vi "getTSRnumber.vi"(8 "error in (no error)":errorcluster, 11 "reference in":refnum<class "File Controller.lvclass">) -> (0 "error out":errorcluster, 3 "reference out":refnum<class "File Controller.lvclass">)   [LabVIEW 2016, in "File Controller.lvclass"]
uses:
  File Controller.lvclass
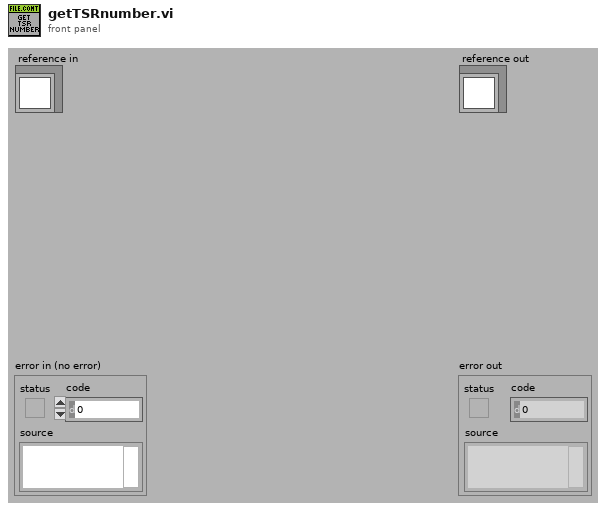
[diagram p1: front panel]
types:
  T1 = typedef "File Controller.lvclass/ObjectAttributesRef.ctl" = refnum<data-value>
  T2 = typedef "File Controller.lvclass/ObjectAttributes.ctl" = cluster{"MyAttribute":dbl, "excelFile_refs":refnum<class "excelFile.lvclass">[], "filePaths":path[], "outlookTemplatePaths":path[], "attachmentTemplatePaths":path[], "configFilePath":path, "not_setting":bool[], "python_ref":refnum<class "python.lvclass">, "TSR":cluster{"number":string, "TSR_path":path, "service_path":path, "email_to":string}}
  T3 = cluster{"number":string, "TSR_path":path, "service_path":path, "email_to":string}
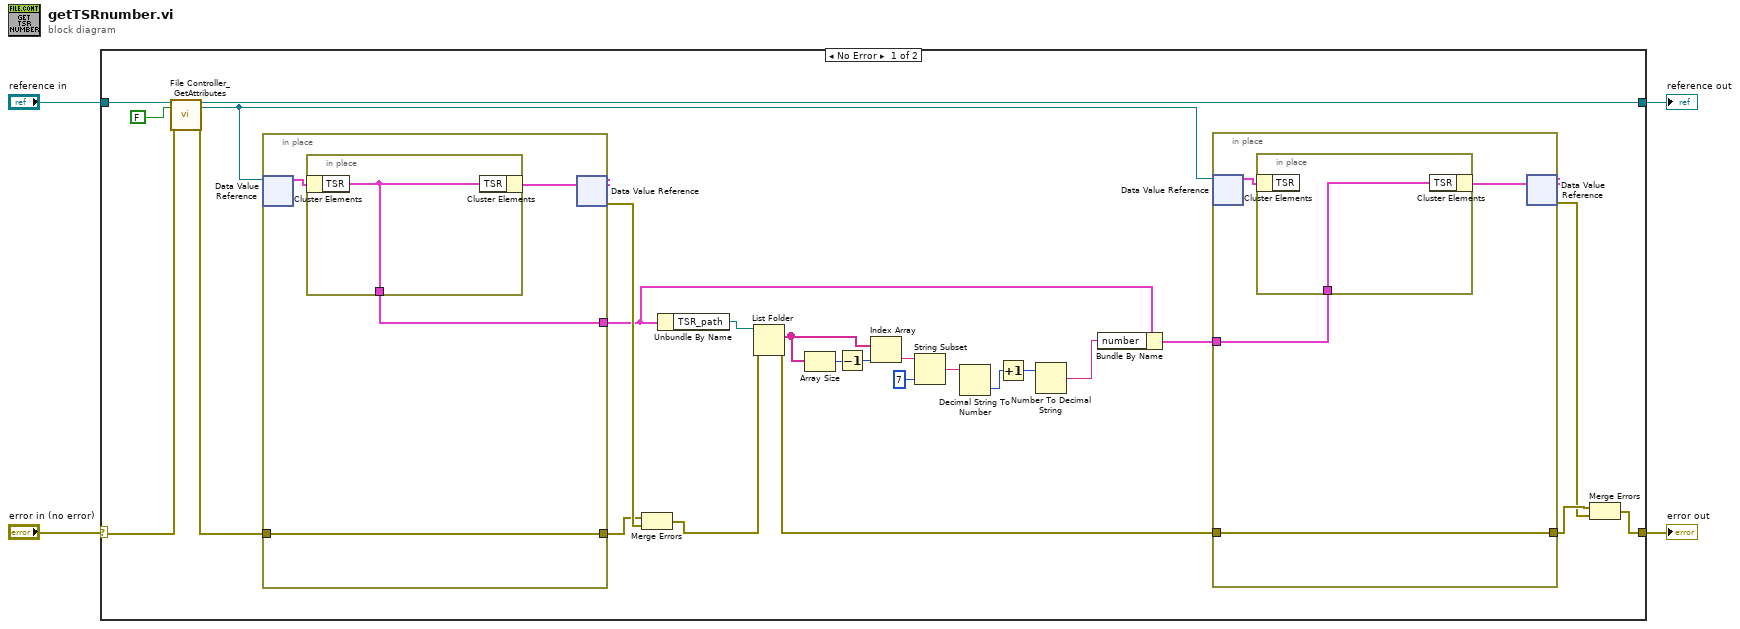
[diagram p0: block diagram]
diagram:
  n1 = case shown="No Error" "error in (no error)" {
    selector: "error in (no error)" -> [w25 w41]
    tunnel: [w9 w41] -> w3
    tunnel: [w23 w40] -> w1
    tunnel: "reference in" -> [w27 w40]
    frame No Error {
      n2 = call "File Controller_GetAttributes.vi"("reference in"=w27, "return data? (T)"=FALSE, "error in (no error)"=w25) -> ("reference out"=w23:refnum<class "File Controller.lvclass">, "attributes ref"=w13:T1, "error out"=w24:errorcluster)  [unwired: 13 in, 1 out]
      n3 = in-place {
        in-place-border: w24 -> [w36]
        in-place-border: [w36] -> w28
        in-place-border: [w35] -> w15
        n4 = in-place-dvr #1(w13) -> (w37:T2)  [unwired: 1 out]
        n5 = in-place {
          in-place-border: [w39] -> w35
          n6 = in-place-cluster #2(w37) -> ("TSR"=w39:T3)
          n7 = in-place-cluster #2("TSR"=w39) -> (w38:T2)
        }
        n8 = in-place-dvr #1(w38) -> (w29:errorcluster)  [unwired: 1 out]
      }
      n9 = Merge Errors(w28, w29) -> (w21:errorcluster)
      n10 = Unbundle By Name(w15) -> ("TSR_path"=w22:path)
      n11 = List Folder(path=w22, error in=w21) -> (filenames=w20:string[], error out=w14:errorcluster)  [unwired: 2 in, 2 out]
      n12 = Array Size(array=w20) -> (size(s)=w19:i32)
      n13 = Decrement(x=w19) -> (x-1=w18:i32)
      n14 = Index Array(array=w20, index=w18) -> (element=w17:string)
      n15 = String Subset(string=w17, length (rest)=7 ("length (rest)")) -> (substring=w8:string)  [unwired: 1 in]
      n16 = Decimal String To Number(string=w8) -> (number=w7:i32)  [unwired: 2 in, 1 out]
      n17 = Increment(x=w7) -> (x+1=w5:i32)
      n18 = Number To Decimal String(number=w5) -> (decimal integer string=w6:string)  [unwired: 1 in]
      n19 = Bundle By Name(cluster=w15, "number"=w6) -> (w12:T3)
      n20 = in-place {
        in-place-border: w14 -> [w31]
        in-place-border: [w31] -> w11
        in-place-border: w12 -> [w30]
        n21 = in-place-dvr #3(w13) -> (w32:T2)  [unwired: 1 out]
        n22 = in-place {
          in-place-border: w30 -> [w34]
          n23 = in-place-cluster #4(w32) -> ()  [unwired: 1 out]
          n24 = in-place-cluster #4("TSR"=w34) -> (w33:T2)
        }
        n25 = in-place-dvr #3(w33) -> (w10:errorcluster)  [unwired: 1 out]
      }
      n26 = Merge Errors(w11, w10) -> (w9:errorcluster)
    }
    frame Error {
    }
  }
  "error out" <- w3
  "reference out" <- w1
